vi "set_power.vi"(8 "error in (no error)":errorcluster, 10 "power in":dbl[unit], 11 "LightSourceMH110125Tsunami in":refnum<class "LightSourceMH110125Tsunami.lvclass">) -> (0 "error out":errorcluster, 3 "LightSourceMH110125Tsunami out":refnum<class "LightSourceMH110125Tsunami.lvclass">)   [LabVIEW 2010, in "LightSourceMH110125Tsunami.lvclass"]
uses:
  LightSourceMH110125Tsunami.lvclass
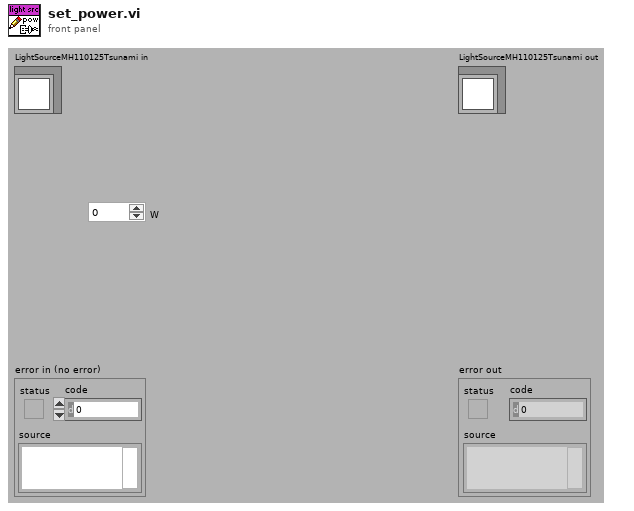
[diagram p1: front panel]
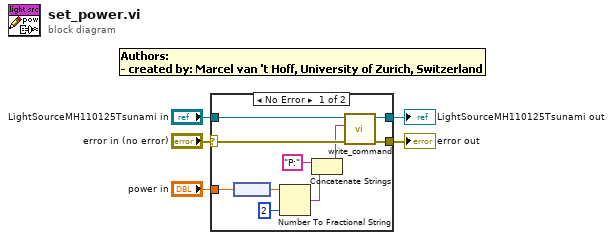
[diagram p0: block diagram]
diagram:
  n1 = case shown="No Error" "error in (no error)" {
    selector: "error in (no error)" -> [w15 w17]
    tunnel: [w14 w17] -> w4
    tunnel: [w12 w16] -> w2
    tunnel: "LightSourceMH110125Tsunami in" -> [w13 w16]
    tunnel: "power in" -> [w9 _]
    frame No Error {
      n2 = node(w9) -> (w10:dbl)
      n3 = Number To Fractional String(number=w10, precision (6)=i16 2) -> (F-format string=w7:string)  [unwired: 2 in]
      n4 = Concatenate Strings("P:" ("string"), w7) -> (w6:string)
      n5 = call-dynamic "write_command.vi"("error in (no error)"=w15, "string to write"=w6, "LightSourceMH110125Tsunami in"=w13) -> ("error out"=w14:errorcluster, "LightSourceMH110125Tsunami out"=w12:refnum<class "LightSourceMH110125Tsunami.lvclass">)  [unwired: 6 in, 1 out]
    }
    frame Error {
    }
  }
  "error out" <- w4
  "LightSourceMH110125Tsunami out" <- w2
